vi "CC Observation Generate Filter Wheel Step.vi"(8 "error in (no error)":errorcluster, 10 "Wheel (0 or 1)":i32, 11 "Filter Wheel Name":string) -> (0 "error out":errorcluster, 3 "Step":T1={"Action"=enum."Acquire Images", "Data"=variant})   [LabVIEW 2021]
uses:
  typedefs/CC Script Step.ctl
  typedefs/CC enum Script Action.ctl
  typedefs/CC cluster Filter Wheel Parameters.ctl
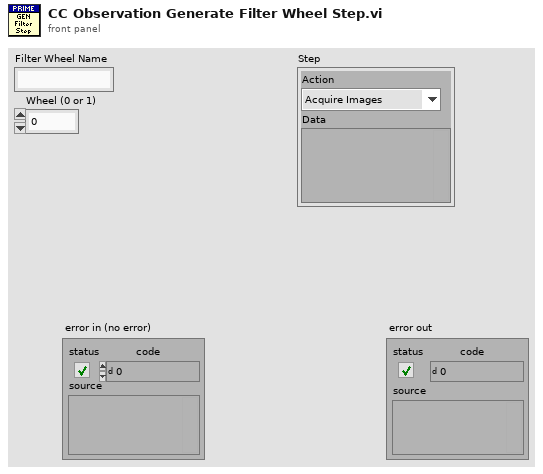
[diagram p1: front panel]
types:
  T1 = typedef "CC Script Step.ctl" = cluster{"Action":T2, "Data":variant}
  T2 = typedef "CC enum Script Action.ctl" = enum16{"Noop", "Define Object", "Define Exposure", "Define Dithering", "Acquire Images", "Set Filter Wheel", "Telescope Home", "Telescope Move", "Telescope RA DEC", "Focus Move Relative", "Focus Move Absolute", "Focus Set Home", "Macro", "Pause", "Ask User", "Define Random Dither"}
  T3 = typedef "CC cluster Filter Wheel Parameters.ctl" = cluster{"Wheel":i32, "Filter":i32}
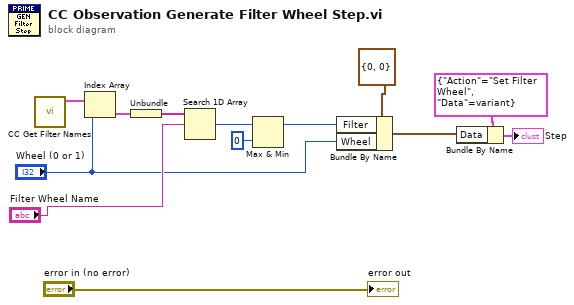
[diagram p0: block diagram]
diagram:
  n1 = call "CC Get Filter Names.vi"() -> ("filter names"=w11:cluster{"Names":string[]}[])  [unwired: 9 in, 2 out]
  n2 = Index Array(array=w11, index="Wheel (0 or 1)") -> (element=w8:cluster{"Names":string[]})
  n3 = Unbundle(w8) -> ("Names"=w10:string[])
  n4 = Search 1D Array(1D array=w10, element="Filter Wheel Name") -> (index of element=w9:i32)  [unwired: 1 in]
  n5 = Max & Min(x=w9, y=0) -> (max(x,y)=w5:i32)  [unwired: 1 out]
  n6 = Bundle By Name(cluster=T3 {"Wheel"=0, "Filter"=0} ("Acquire Parameters in"), "Filter"=w5, "Wheel"="Wheel (0 or 1)") -> (w2:T3)
  n7 = Bundle By Name(cluster=T1 {"Action"=enum."Set Filter Wheel", "Data"=variant} ("Cluster"), "Data"=w2) -> (→"Step":T1)
  "error out" <- "error in (no error)"
